vi "Butterfly_extract_VPI_VRL - HLH.vi"(9 "Threshold":dbl, 10 "Voltage Array":dbl[](array[numeric]), 11 "Result Array In":dbl[][](array[numeric])) -> (2 "VRLs":dbl[](array[numeric]), 3 "VPIs":dbl[](array[numeric]))   [LabVIEW 2013]
doc: "Extracts the VPI and VRL with respect to the given threshold for a data set that starts high value, goes below threshold, and comes back above the threshold (HLH)."
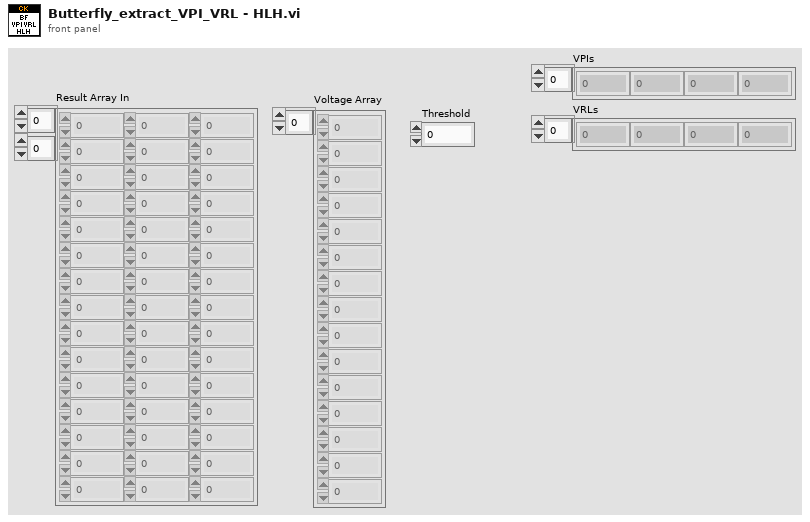
[diagram p1: front panel]
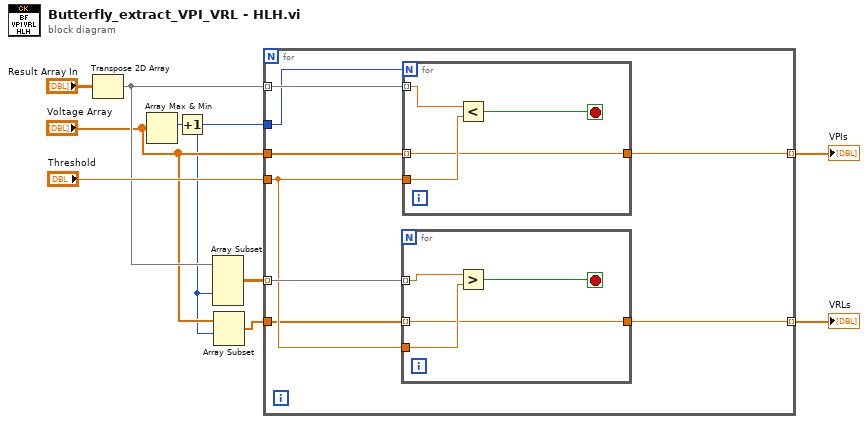
[diagram p0: block diagram]
diagram:
  n1 = Transpose 2D Array(2D array="Result Array In") -> (transposed array=w4:dbl[][])
  n2 = Array Max & Min(array="Voltage Array") -> (max index (indices)=w8:i32)  [unwired: 3 out]
  n3 = Increment(x=w8) -> (x+1=w1:i32)
  n4 = Array Subset(array=w4, index (col)=w1) -> (w7:dbl[][])  [unwired: 3 in]
  n5 = Array Subset(array="Voltage Array", index=w1) -> (w3:dbl[])  [unwired: 1 in]
  n6 = for {
    tunnel: w4 -> [w13] mode=indexing
    tunnel: "Threshold" -> [w16]
    tunnel: [w18] -> w9 mode=indexing
    tunnel: w1 -> [w12]
    tunnel: "Voltage Array" -> [w15]
    tunnel: w7 -> [w17] mode=indexing
    tunnel: [w14] -> w6 mode=indexing
    tunnel: w3 -> [w11]
    n7 = for {
      tunnel: w17 -> [w22] mode=indexing
      tunnel: w16 -> [w21]
      tunnel: w11 -> [w19] mode=indexing
      tunnel: [w19] -> w14
      stop <- w20 stop-if-true
      n8 = Greater?(x=w22, y=w21) -> (0:w20:bool)
    }
    n9 = for {
      N: w12 -> [_]
      tunnel: w13 -> [w26] mode=indexing
      tunnel: w16 -> [w25]
      tunnel: w15 -> [w23] mode=indexing
      tunnel: [w23] -> w18
      stop <- w24 stop-if-true
      n10 = Less?(x=w26, y=w25) -> (x < y?=w24:bool)
    }
  }
  "VPIs" <- w9
  "VRLs" <- w6
